vi "Set_Parameter_Instrument (Json).vi"(8 "error in (no error)":errorcluster caption="entrée d'erreur (pas d'erreur)", 10 "Parameter (Json)":string, 11 "Flash_Jlink en entrée":refnum<class "Flash_STM32.lvclass">) -> (0 "error out":errorcluster caption="sortie d'erreur", 3 "Flash_Jlink en sortie":refnum<class "Flash_STM32.lvclass">)   [LabVIEW 2020, in "Library Test.lvlib" / "Flash_STM32.lvclass"]
uses:
  Flash_STM32.lvclass
  C:/Users/ngarcin/OneDrive - Altyor/Standard TB/Class/Test/Test (Default)/Test (Default).lvclass
  Commun VI/TypeDef/Commande Test/Commande Parameter Flash_STM32.ctl
  Flash_STM32.lvclass/Flash_STM32.ctl
  JSON API/JSON Value/Set from JSON string.vi
  Test_Without_Instr/Test_Without_Inst.lvclass
  JSON API/JSON Value/JSON Value.lvclass
  JSON API/Variant JSON/Variant JSON.lvlib
  JSON API/Get Polymorphic/JSON GetSet.lvlib
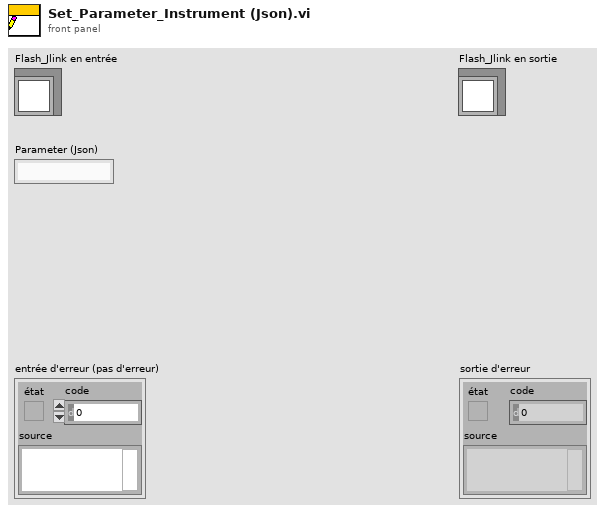
[diagram p1: front panel]
types:
  T1 = typedef "Commande Parameter Flash_STM32.ctl" = cluster{"Path FW":path, "Working Directory":path, "Connection_Type":string}
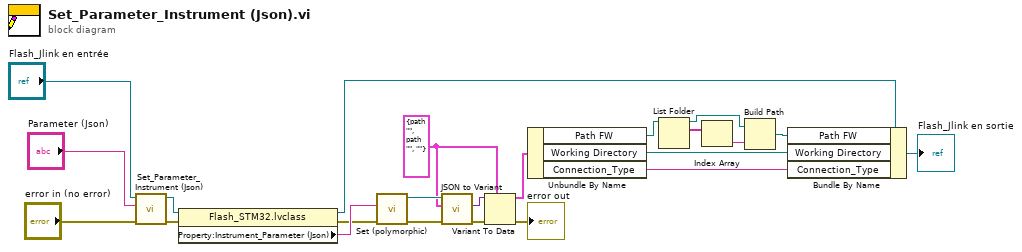
[diagram p0: block diagram]
diagram:
  w2 = T1 {"Path FW"=path "", "Working Directory"=path "", "Connection_Type"=""} ("Cluster")
  n1 = call-parent "Set_Parameter_Instrument (Json).vi"("error in (no error)"="error in (no error)", "Parameter (Json)"="Parameter (Json)", "Test (Default) en entrée"="Flash_Jlink en entrée") -> ("error out"=w13:errorcluster, "Test (Default) en sortie"=w15:refnum<class "Flash_STM32.lvclass">)  [unwired: 7 in]
  n2 = property class="Flash_STM32.lvclass"(reference=w15, error in=w13) -> (reference out=w12:refnum<class "Flash_STM32.lvclass">, error out=w10:errorcluster, "Property:Instrument_Parameter (Json)"=w14:string)
  n3 = call-poly "Set (polymorphic).vi"("error in (no error)"=w10, "JSON stream"=w14) -> ("error out"=w17:errorcluster, "JSON Value out"=w19:refnum<class "JSON Value.lvclass">)  [unwired: 7 in, 1 out]
  n4 = call "JSON to Variant.vi"("error in (no error)"=w17, "Variant (Data Type)"=w2, "JSON Value"=w19) -> ("error out"=w18:errorcluster, "Variant out"=w16:variant)  [unwired: 7 in]
  n5 = Variant To Data(error in=w18, type=w2, Variant=w16) -> (data=w11:T1, error out=→"error out":errorcluster)
  n6 = Unbundle By Name(w11) -> ("Path FW"=w4:path, "Working Directory"=w8:path, "Connection_Type"=w1:string)
  n7 = List Folder(path=w4) -> (path out=w5:path, filenames=w7:string[])  [unwired: 3 in, 2 out]
  n8 = Index Array(array=w7) -> (element=w6:string)  [unwired: 1 in]
  n9 = Build Path(base path=w5, name or relative path=w6) -> (appended path=w3:path)
  n10 = Bundle By Name(cluster=w12, "Path FW"=w3, "Working Directory"=w8, "Connection_Type"=w1) -> (→"Flash_Jlink en sortie":refnum<class "Flash_STM32.lvclass">)
